vi "InterfaceCasting.vi"() -> ()   [LabVIEW 2016]
panel:
  out "EscapedMode":i32
  in  "ActiveDs.IADsADSystemInfo":refnum<k7>
  in  "ActiveDs.IADsPathname":refnum<k7>
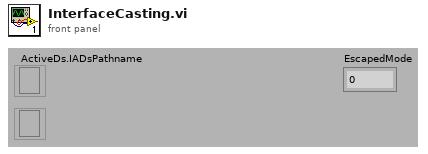
[diagram p1: front panel]
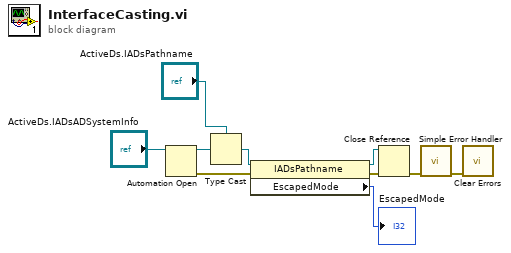
[diagram p0: block diagram]
diagram:
  n1 = Automation Open(Automation Refnum="ActiveDs.IADsADSystemInfo") -> (Automation Refnum=w2:refnum<k7>, error out=w3:errorcluster)  [unwired: 1 in, 2 out]
  n2 = Type Cast(type="ActiveDs.IADsPathname", x=w2) -> (*(type *) &x=w1:refnum<k7>)
  n3 = property class="IADsPathname"(reference=w1, error in=w3) -> (reference out=w9:refnum<k7>, error out=w10:errorcluster, "EscapedMode"=→"EscapedMode":i32)
  n4 = Close Reference(reference=w9, error in (no error)=w10) -> (error out=w8:errorcluster)
  n5 = call <vilib>:"Simple Error Handler.vi"("error in (no error)"=w8) -> ("error out"=w7:errorcluster)  [unwired: 1 in, 7 out]
  n6 = call <vilib>:"Clear Errors.vi"("error in (no error)"=w7) -> ()  [unwired: 1 in, 6 out]
